vi "adaptPosEstBall.vi"(4 "AttakingOurselves":bool, 6 "Utilities.lvclass":refnum<class "Utilities.lvclass">, 8 "error in (no error)":errorcluster, 9 "Robot":refnum<class "Robot.lvclass">, 10 "BallRef":refnum<class "Ball.lvclass">, 11 "KickToSkill in":refnum<class "KickToSkill.lvclass">) -> (0 "error out":errorcluster, 2 "Pos_est adapted":dbl[](array[numeric]), 3 "KickToSkill out":refnum<class "KickToSkill.lvclass">)   [LabVIEW 2021, in "KickToSkill.lvclass"]
uses:
  KickToSkill.lvclass
  Ball_class/Ball.lvclass
  D:/RoboIme/horie/SSL_AI/Object_class/Object.lvclass
  Robot_class/Robot.lvclass
  Utilities_class/Utilities.lvclass
  Ball_class/Ball.lvclass/Ball.ctl
  Object_class/Object.lvclass/Object.ctl
  <vilib>/Analysis/_algsub.llb/Real Vector Norm.vi
  Object_class/Read x.vi
  Object_class/Read y.vi
  Ball_class/Read v_x.vi
  Ball_class/Read v_y.vi
  Object_class/Read pos_est_x.vi
  Object_class/Read pos_est_y.vi
  <vilib>/Analysis/NI_AALPro.lvlib
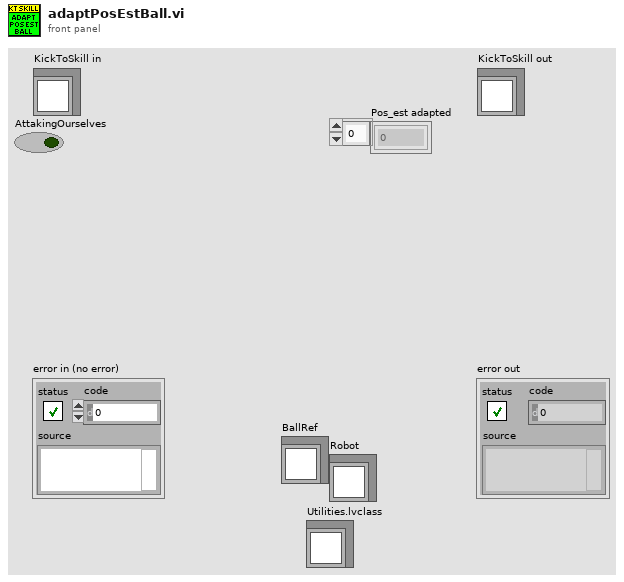
[diagram p1: front panel]
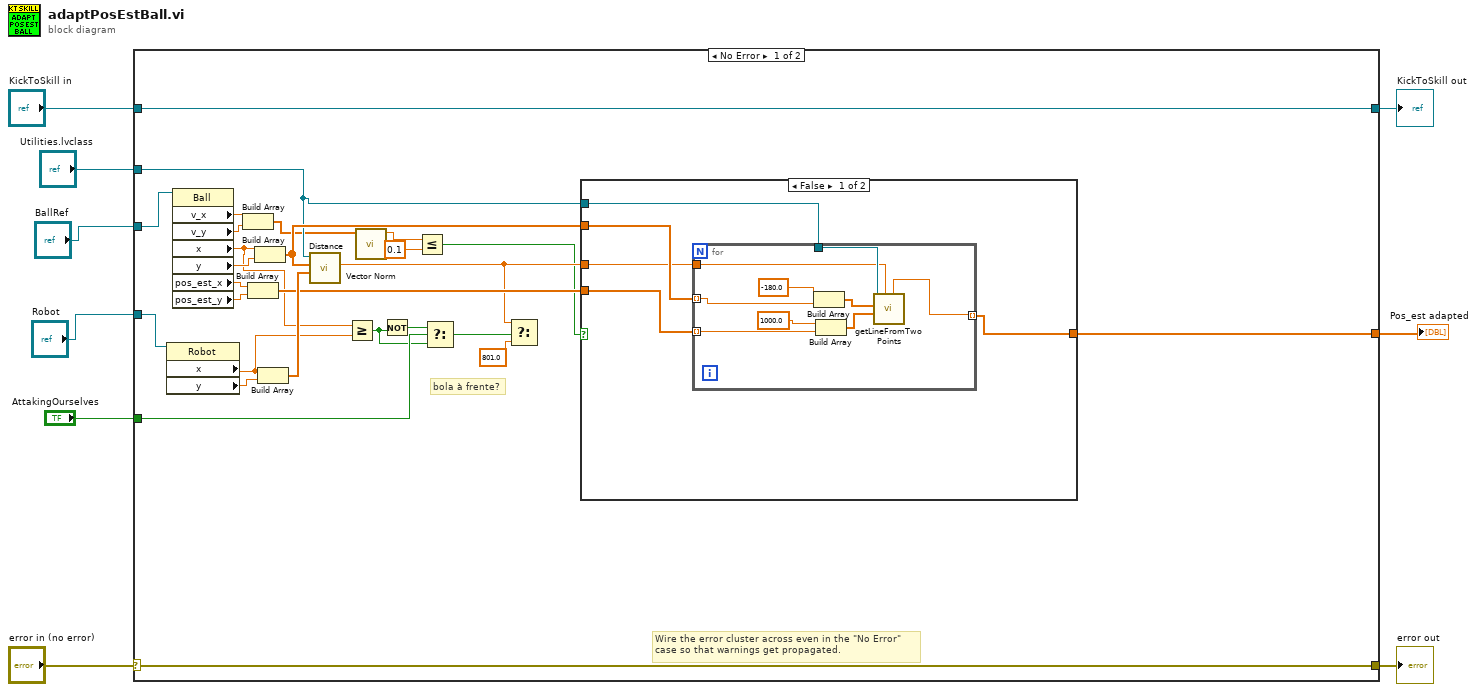
[diagram p0: block diagram]
diagram:
  n1 = case shown="No Error" "error in (no error)" {
    selector: "error in (no error)" -> [w35 w53]
    tunnel: [w35 w53] -> w8
    tunnel: [w36 w52] -> w6
    tunnel: "KickToSkill in" -> [w36 w52]
    tunnel: "BallRef" -> [w34 _]
    tunnel: "Robot" -> [w33 _]
    tunnel: "Utilities.lvclass" -> [w24 _]
    tunnel: [w29 _] -> w2
    tunnel: "AttakingOurselves" -> [w19 _]
    frame No Error {
      # "bola à frente?"
      # "Wire the error cluster across even in the \"No Error\"\ncase so that warnings get propagated."
      n2 = property class="Robot"(reference=w33) -> ("x"=w22:dbl, "y"=w31:dbl)  [unwired: 1 in, 2 out]
      n3 = property class="Ball"(reference=w34) -> ("v_x"=w15:dbl, "v_y"=w14:dbl, "x"=w23:dbl, "y"=w32:dbl, "pos_est_x"=w27:dbl, "pos_est_y"=w26:dbl)  [unwired: 1 in, 2 out]
      n4 = Build Array(w15, w14) -> (w13:dbl[])
      n5 = Build Array(w27, w26) -> (w25:dbl[])
      n6 = Build Array(w23, w32) -> (w28:dbl[])
      n7 = Build Array(w22, w31) -> (w30:dbl[])
      n8 = call "Distance.vi"("P1"=w30, "P2"=w28, "Utilities in"=w24) -> ("Distance"=w21:dbl)  [unwired: 6 in, 2 out]
      n9 = Greater Or Equal?(x=w23, y=w22) -> (x >= y?=w18:bool)
      n10 = call-poly <vilib>:"Vector Norm.vi"("Input Vector"=w13) -> ("norm"=w12:dbl)  [unwired: 9 in, 1 out]
      n11 = Not(x=w18) -> (.not. x?=w17:bool)
      n12 = Less Or Equal?(x=w12, y=0.1) -> (x <= y?=w10:bool)
      n13 = Select(t=w17, s=w19, f=w18) -> (s? t:f=w16:bool)
      n14 = Select(t=w21, s=w16, f=801.0) -> ()  [unwired: 1 out]
      n15 = case shown="False" w10 {
        tunnel: [w41 w51] -> w29
        tunnel: w28 -> [w40 w51]
        tunnel: w25 -> [w39 _]
        tunnel: w24 -> [w38 _]
        tunnel: w21 -> [w37 _]
        frame False {
          n16 = for {
            tunnel: w38 -> [w50]
            tunnel: w40 -> [w47] mode=indexing
            tunnel: w39 -> [w46] mode=indexing
            tunnel: w37 -> [w43]
            tunnel: [w42] -> w41 mode=indexing
            n17 = Build Array(-180.0, w47) -> (w45:dbl[])
            n18 = Build Array(1000.0, w46) -> (w44:dbl[])
            n19 = call "getLineFromTwoPoints.vi"("x informed (optional)"=w43, "Point 2"=w44, "Point 1"=w45, "Utilities in"=w50) -> ("y to x informed (opitional)"=w42:dbl)  [unwired: 3 in, 4 out]
          }
        }
        frame True {
        }
      }
    }
    frame Error {
    }
  }
  "error out" <- w8
  "KickToSkill out" <- w6
  "Pos_est adapted" <- w2
